vi "Write Error.vi"(8 "error in":errorcluster, 11 "connection info in":T1) -> (0 "error out":errorcluster, 3 "connection info out":T1)   [LabVIEW 2010, in "NI_CCC.lvlib"]
uses:
  NI_CCC.lvlib
  <vilib>/NI/STM/TCP/TCP Connection Info.ctl
  <vilib>/NI/STM/SubVIs/MetaDataElement.ctl
  <vilib>/NI/STM/TCP/TCP Write Options.ctl
  <vilib>/NI/STM/NI STM.lvlib
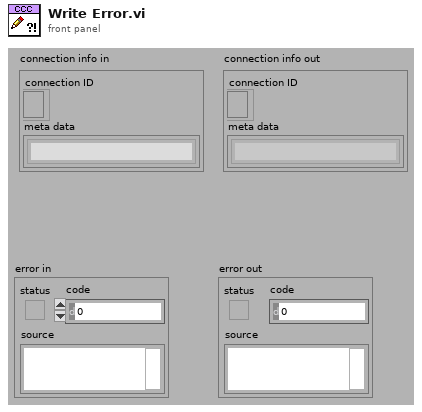
[diagram p1: front panel]
types:
  T1 = typedef "NI STM.lvlib/TCP Connection Info.ctl" = cluster{"connection ID":refnum<k5>, "meta data":T2[]}
  T2 = typedef "NI STM.lvlib/MetaDataElement.ctl" = string
  T3 = typedef "NI STM.lvlib/TCP Write Options.ctl" = cluster{"ignore timeout error":bool, "timeout ms (1000)":i32}
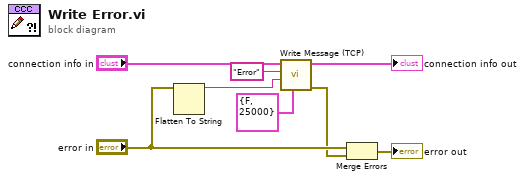
[diagram p0: block diagram]
diagram:
  n1 = Flatten To String(anything="error in") -> (data string=w5:string)  [unwired: 1 in, 4 out]
  n2 = call <vilib>:"Write Message (TCP).vi"("options"=T3 {"ignore timeout error"=FALSE, "timeout ms (1000)"=25000} ("Options"), "data"=w5, "name"="Error" ("Name"), "connection info in"="connection info in") -> ("error out"=w2:errorcluster, "connection info out"=→"connection info out":T1)  [unwired: 6 in]
  n3 = Merge Errors("error in", w2) -> (→"error out":errorcluster)
